vi "Centroid.vi"(10 "Points":refnum<class "Vec3d Class.lvclass">[](array[class])) -> (2 "Centroid":refnum<class "Vec3d Class.lvclass">)   [LabVIEW 2011]
uses:
  Vec3d Class/Vec3d Class.lvclass
  <vilib>/Analysis/NI_AALBase.lvlib
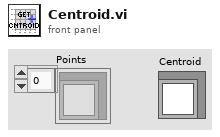
[diagram p1: front panel]
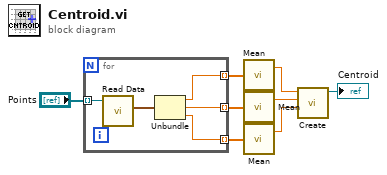
[diagram p0: block diagram]
diagram:
  n1 = for {
    tunnel: "Points" -> [w13] mode=indexing
    tunnel: [w11] -> w6 mode=indexing
    tunnel: [w10] -> w5 mode=indexing
    tunnel: [w9] -> w7 mode=indexing
    n2 = call-dynamic "Read Data.vi"("Vec3d Class in"=w13) -> ("Data"=w12:cluster{"X":dbl, "Y":dbl, "Z":dbl})  [unwired: 8 in, 2 out]
    n3 = Unbundle(w12) -> ("X"=w11:dbl, "Y"=w10:dbl, "Z"=w9:dbl)
  }
  n4 = call <vilib>:"Mean.vi"("X"=w6) -> ("mean"=w4:dbl)  [unwired: 1 out]
  n5 = call <vilib>:"Mean.vi"("X"=w5) -> ("mean"=w3:dbl)  [unwired: 1 out]
  n6 = call <vilib>:"Mean.vi"("X"=w7) -> ("mean"=w2:dbl)  [unwired: 1 out]
  n7 = call "Create.vi"("Z"=w2, "Y"=w3, "X"=w4) -> ("Vec3d Class out"=→"Centroid":refnum<class "Vec3d Class.lvclass">)  [unwired: 7 in, 1 out]
